vi "Send_Data.vi"(1 "Upload to pc cycle":i32, 2 "Counter":i32) -> (0 "value":dbl)   [LabVIEW 2017]
uses:
  <vilib>/myRIO/Instrument Drivers/Onboard IO/AI/typedefs/AI Reference.ctl
  <vilib>/myRIO/Common/Instrument Driver Framework/Utilities/typedefs/myRIO Generic Hardware Reference.ctl
  <vilib>/myRIO/Common/Instrument Driver Framework/Utilities/typedefs/Hardware Version Enum.ctl
  <vilib>/myRIO/Common/Instrument Driver Framework/Utilities/typedefs/myRIO v1.0 Reference.ctl
  <vilib>/myRIO/Common/Instrument Driver Framework/Utilities/typedefs/Generic FPGA Reference.ctl
  <vilib>/myRIO/Common/Instrument Driver Framework/myRIO v1.0/AI/typedefs/AI Channels List.ctl
  <vilib>/myRIO/Common/Instrument Driver Framework/myRIO v1.0/AI/typedefs/AI Channels Enum.ctl
  <vilib>/myRIO/Common/Instrument Driver Framework/Utilities/typedefs/Analog Scaling Constants List.ctl
  <vilib>/myRIO/Common/Instrument Driver Framework/Utilities/typedefs/Analog Scaling Constants.ctl
  <vilib>/userdefined/High Color/nirio_resource_hc.ctl
  Bundle_array.ctl
  <vilib>/myRIO/Common/Instrument Driver Framework/Utilities/vis/Is FPGA Ref Available.vi
  <vilib>/myRIO/Common/Instrument Driver Framework/myRIO v1.0/AI/vis/myRIO v1.1 Open AI.vi
  <vilib>/myRIO/Instrument Drivers/Onboard IO/AI/vis/Read.vi
  <vilib>/myRIO/Common/Instrument Driver Framework/Utilities/vis/Validate Channels.vi
  <vilib>/myRIO/Common/Instrument Driver Framework/myRIO v1.0/AI/vis/myRIO v1.0 Reserve AI.vi
  <vilib>/myRIO/Common/Instrument Driver Framework/myRIO v1.0/AI/vis/myRIO v1.0 Build MUX Configuration AI.vi
  <vilib>/myRIO/Common/Instrument Driver Framework/myRIO v1.0/Resource Manager/vis/myRIO v1.0 Reserve Channel List.vi
  <vilib>/myRIO/Common/Instrument Driver Framework/myRIO v1.0/Resource Manager/vis/myRIO v1.0 Reserve Channel.vi
  <vilib>/myRIO/Common/Instrument Driver Framework/myRIO v1.0/Resource Manager/vis/myRIO v1.0 Unreserve Channel.vi
  <vilib>/myRIO/Common/Instrument Driver Framework/myRIO v1.0/Resource Manager/vis/myRIO v1.0 Build Mutex Name.vi
  <vilib>/Utility/VariantDataType/GetNumericInfo.vi
  <vilib>/Utility/error.llb/Error Cluster From Error Code.vi
  <vilib>/myRIO/Common/Instrument Driver Framework/myRIO v1.0/myRIO v1.1 Open.vi
  <vilib>/myRIO/Common/Instrument Driver Framework/myRIO v1.0/AI/vis/myRIO v1.0 Get Scaling Constants AI.vi
  <vilib>/myRIO/Common/Instrument Driver Framework/Utilities/vis/IO Manager.vi
  <vilib>/myRIO/Common/Instrument Driver Framework/Utilities/vis/Configuration Manager.vi
  <vilib>/myRIO/Common/Instrument Driver Framework/myRIO v1.0/myRIO v1.0 Close.vi
  <vilib>/myRIO/Common/Instrument Driver Framework/myRIO v1.0/AI/vis/myRIO v1.0 Read AI.vi
  <vilib>/myRIO/Express VI/Onboard IO/AI/AI Express VI.xnode
  <vilib>/myRIO/Instrument Drivers/Onboard IO/AI/vis/myRIO AI Open.xnode
  <vilib>/myRIO/Instrument Drivers/Onboard IO/AI/AI.lvlib
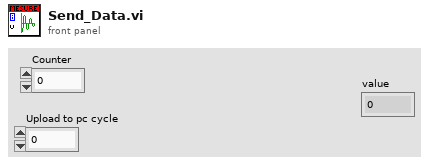
[diagram p1: front panel]
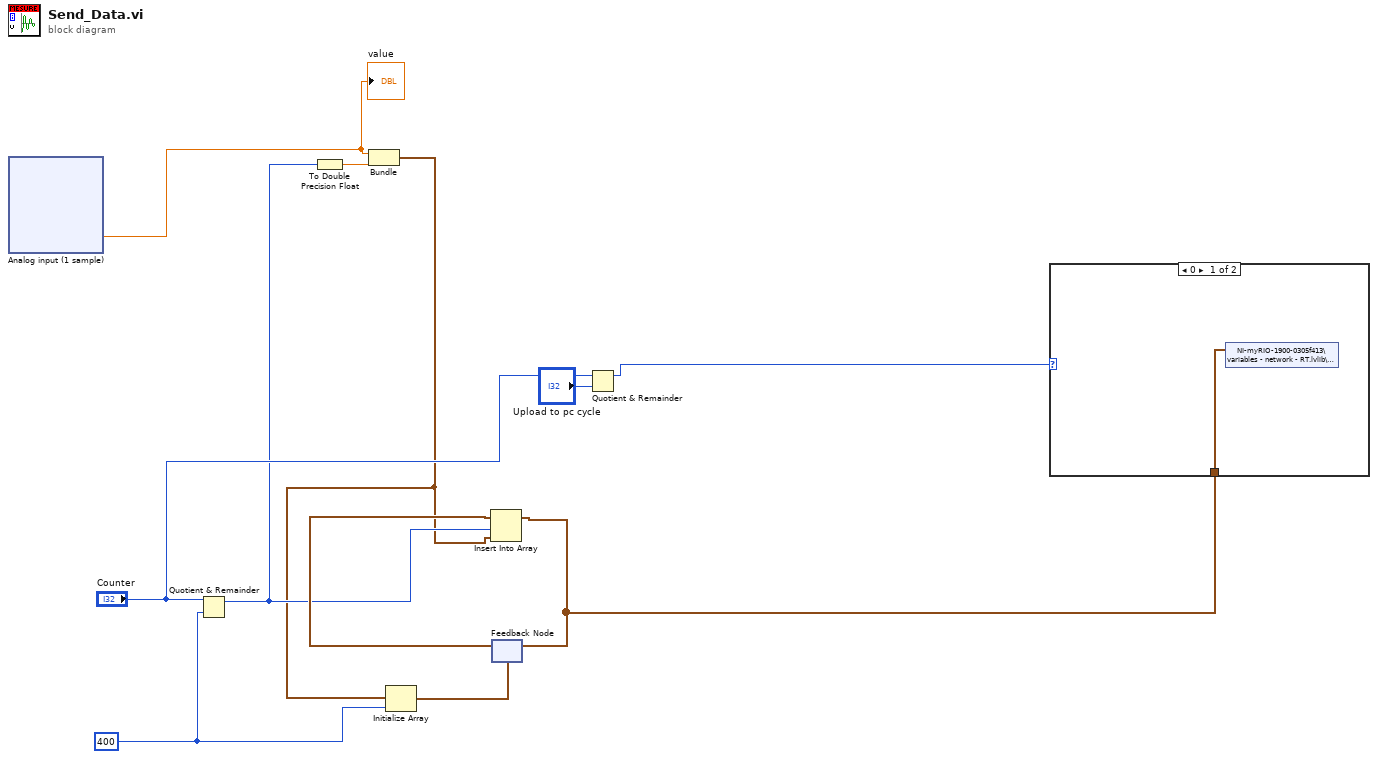
[diagram p0: block diagram]
diagram:
  w9 = 400 ("dimension size")
  n1 = xnode "Analog input (1 sample)"() -> ("distance (C/AI0 (AI0))"=w1:dbl)  [unwired: 1 in, 1 out]
  "value" <- w1
  n2 = Quotient & Remainder(x="Counter", y=w9) -> (x-y*floor(x/y)=w3:i32)  [unwired: 1 out]
  n3 = To Double Precision Float(number=w3) -> (double precision float=w4:dbl)
  n4 = Bundle("distance (C/AI0 (AI0))"=w1, w4) -> (w2:cluster{"distance (C/AI0 (AI0))":dbl, dbl})  [unwired: 1 in]
  n5 = Initialize Array(w2, w9) -> (w11:cluster{"distance (C/AI0 (AI0))":dbl, dbl}[])
  n6 = feedback #1(w11) -> (w10:cluster{"distance (C/AI0 (AI0))":dbl, dbl}[])
  n7 = Insert Into Array(array=w10, index=w3, new element=w2) -> (w5:cluster{"distance (C/AI0 (AI0))":dbl, dbl}[])
  n8 = feedback-in #1(w5) -> ()
  n9 = Quotient & Remainder(x="Counter", y="Upload to pc cycle") -> (x-y*floor(x/y)=w7:i32)  [unwired: 1 out]
  n10 = case shown="0" w7 {
    tunnel: w5 -> [w12 _]
    frame 0 {
      n11 = shared-variable "NI-myRIO-1900-0305f413\\variables - network - RT.lvlib\\Bundle_array"(w12) -> ()  [unwired: 1 in, 1 out]
    }
    frame 1, Default {
    }
  }
